vi "ctl activator.vi"(8 "error in":errorcluster, 10 "Disabled":T1(ring), 11 "Array":refnum<vi>[](array[refnum])) -> (0 "error out":errorcluster)   [LabVIEW 2015]
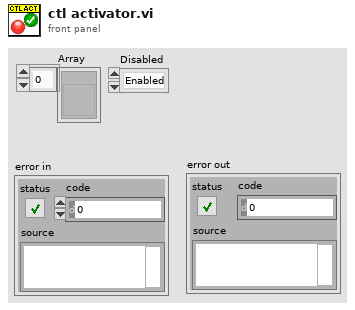
[diagram p1: front panel]
types:
  T1 = enum8{"Enabled", "Disabled", "Disabled and Grayed Out"}
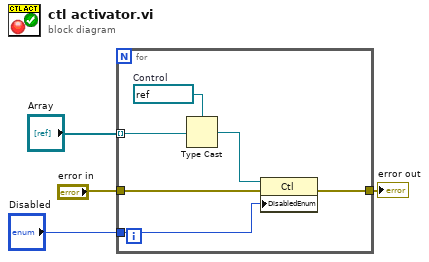
[diagram p0: block diagram]
diagram:
  n1 = for {
    tunnel: "Disabled" -> [w10]
    tunnel: "Array" -> [w7] mode=indexing
    tunnel: [w6] -> w2
    tunnel: "error in" -> [w5]
    w8 = refnum<vi> refnum  # Control
    n2 = Type Cast(type=w8, x=w7) -> (*(type *) &x=w9:refnum<vi>)
    n3 = property class="Ctl"(reference=w9, error in=w5, "DisabledEnum"=w10) -> (error out=w6:errorcluster)  [unwired: 1 out]
  }
  "error out" <- w2
